vi "Transfer Page GUID.vi"() -> (3 "Transfer GUID":string="bcb89113-3f5b-435a-8111-e471fb52bdd7")   [LabVIEW 2019, in "DSF Shared.lvlib"]
uses:
  DSF Shared.lvlib
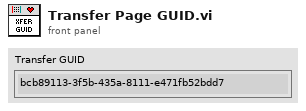
[diagram p1: front panel]
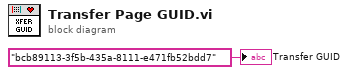
[diagram p0: block diagram]
diagram:
  "Transfer GUID" <- "bcb89113-3f5b-435a-8111-e471fb52bdd7" ("Data Sharing Framework")
